vi "Current Nominal Write.vi"   [LabVIEW 2023, in "Cycler.lvclass"]
uses:
  Cycler.lvclass
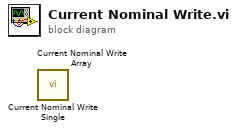
[diagram p0: block diagram]
diagram:
  n1 = call "Current Nominal Write Single.vi"() -> ()  [unwired: 10 in, 2 out]
  n2 = call "Current Nominal Write Array.vi"() -> ()  [unwired: 10 in, 2 out]
